vi "Clustering_Array_Version.vi"(8 "Selected":i64[](array[numeric]), 9 "Inverse_W":dbl[][](array[numeric]) format="%0.3f", 10 "mixing_A":dbl[][](array[numeric]) format="%0.3f", 11 "STFT":dbl[][](array[numeric]) format="%0.3f") -> (0 "TFD Clustering":i32[](array[numeric]), 1 "Z Clustering (KDL)":i32[](array[numeric]), 2 "Z Clustering (EUC)":i32[](array[numeric]), 3 "mixing_A Clustering":i32[](array[numeric]))   [LabVIEW 2014]
uses:
  <vilib>/Analysis/Matrix/Datatypes/RealMatrix.ctl
  <vilib>/Analysis/baseanly.llb/Real A x B.vi
  <vilib>/Analysis/Matrix/Numeric/Conversions/Matrix To Array - RM.vi
  <vilib>/Analysis/NI_AALBase.lvlib
  <vilib>/Analysis/Matrix/NI_Matrix.lvlib
panel:
  out "Centroids of TFD":T1
  out "Centroids of Z (KLD)":T1
  out "Centroids of Z (EUC)":T1
  out "Centroids of Matrix A":T1
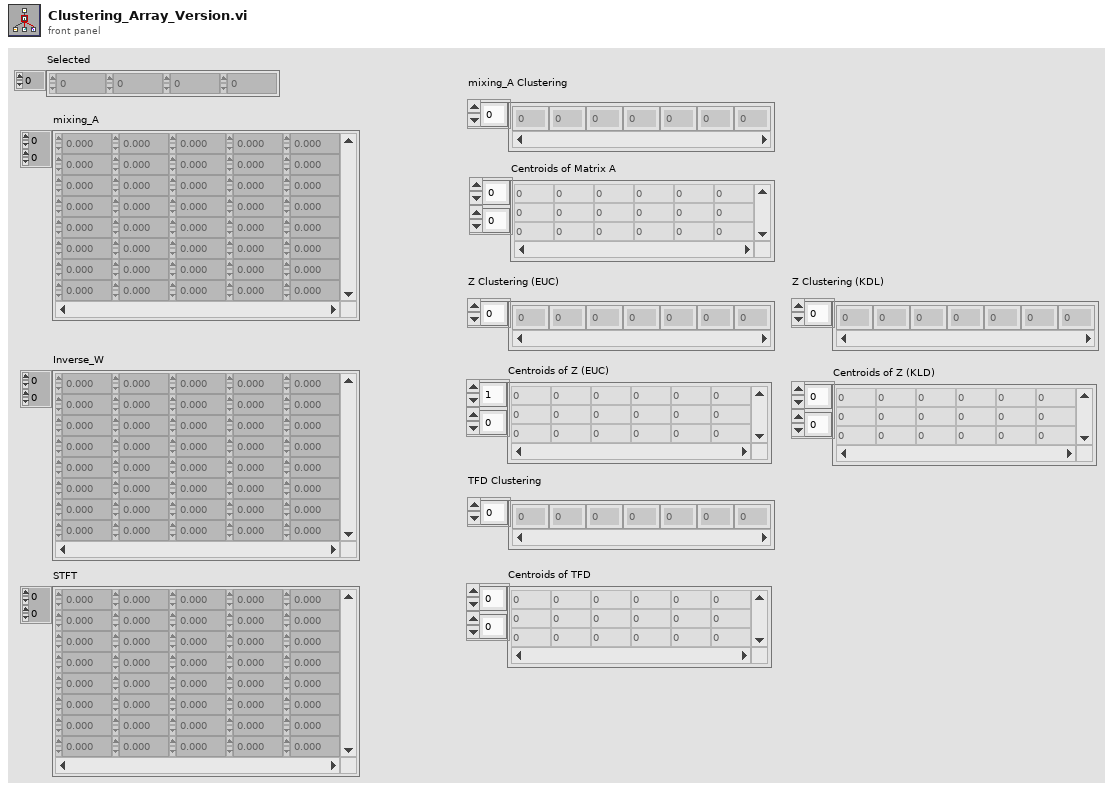
[diagram p1: front panel]
types:
  T1 = typedef "NI_Matrix.lvlib/RealMatrix.ctl" = dbl[][]
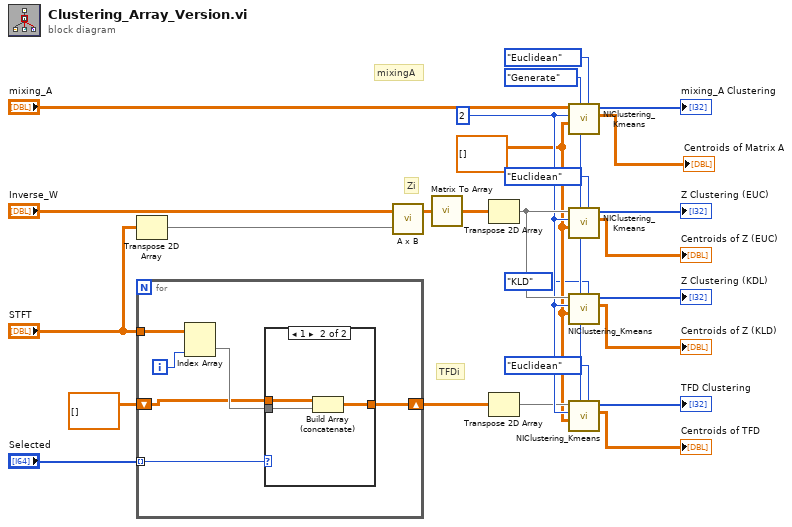
[diagram p0: block diagram]
diagram:
  w17 = dbl[][] [] ("Centroids in")
  w18 = enum16{"Generate", "Input"}."Generate" ("type")
  w20 = 2 ("Classes")
  # "mixingA"
  # "Zi"
  # "TFDi"
  n1 = Transpose 2D Array(2D array="STFT") -> (transposed array=w25:dbl[][])
  n2 = for {
    tunnel: "Selected" -> [w30] mode=indexing
    tunnel: "STFT" -> [w32]
    shift-right: [w28] -> w22
    shift-left: dbl[][] [] -> [w27]
    i -> [w31]
    n3 = Index Array(array=w32, index (col)=w31) -> (element=w29:dbl[])  [unwired: 1 in]
    n4 = case shown="1" w30 {
      tunnel: w29 -> [_ w36]
      tunnel: [w33 w35] -> w28
      tunnel: w27 -> [w33 w34]
      frame 0, Default {
      }
      frame 1 {
        n5 = Build Array (concatenate)(w34, w36) -> (w35:dbl[][])
      }
    }
  }
  n6 = call-poly <vilib>:"A x B.vi"("B"=w25, "A"="Inverse_W") -> ("A x B"=w24:T1)  [unwired: 1 out]
  n7 = call-poly <vilib>:"Matrix To Array.vi"("Real Matrix"=w24) -> ("Real 2D Array"=w23:dbl[][])
  n8 = Transpose 2D Array(2D array=w23) -> (transposed array=w21:dbl[][])
  n9 = Transpose 2D Array(2D array=w22) -> (transposed array=w19:dbl[][])
  n10 = call "NIClustering_Kmeans.vi"("Enum"=enum16{"KLD", "Euclidean"}."Euclidean", "type"=w18, "Centroids in"=w17, "Classes"=w20, "Data"="mixing_A") -> ("Centroids"=→"Centroids of Matrix A":T1, "Results"=→"mixing_A Clustering":i32[])  [unwired: 4 in, 1 out]
  n11 = call "NIClustering_Kmeans.vi"("Enum"=enum16{"KLD", "Euclidean"}."Euclidean", "type"=w18, "Centroids in"=w17, "Classes"=w20, "Data"=w21) -> ("Centroids"=→"Centroids of Z (EUC)":T1, "Results"=→"Z Clustering (EUC)":i32[])  [unwired: 4 in, 1 out]
  n12 = call "NIClustering_Kmeans.vi"("Enum"=enum16{"KLD", "Euclidean"}."KLD", "type"=w18, "Centroids in"=w17, "Classes"=w20, "Data"=w21) -> ("Centroids"=→"Centroids of Z (KLD)":T1, "Results"=→"Z Clustering (KDL)":i32[])  [unwired: 4 in, 1 out]
  n13 = call "NIClustering_Kmeans.vi"("Enum"=enum16{"KLD", "Euclidean"}."Euclidean", "type"=w18, "Centroids in"=w17, "Classes"=w20, "Data"=w19) -> ("Centroids"=→"Centroids of TFD":T1, "Results"=→"TFD Clustering":i32[])  [unwired: 4 in, 1 out]
